vi "_API_BINANCE_GET_SystemStatus.vi"(0 "BinanceAPI in":refnum<class "BinanceAPI_.lvclass">, 11 "error in (no error)":errorcluster) -> (4 "BinanceAPI out":refnum<class "BinanceAPI_.lvclass">, 6 "systemStatus ok? (if True  all work normaly)":bool, 14 "Body":string, 15 "error out":errorcluster)   [LabVIEW 2022 SP3, in "BinanceAPI_.lvclass"]
doc: "https://binance-docs.github.io/apidocs/spot/en/#system-status-system"
uses:
  BinanceAPI_.lvclass
  BinanceAPI_.lvclass/BinanceAPI_.ctl
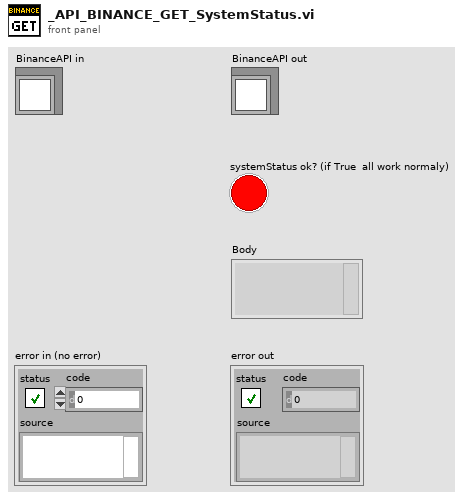
[diagram p1: front panel]
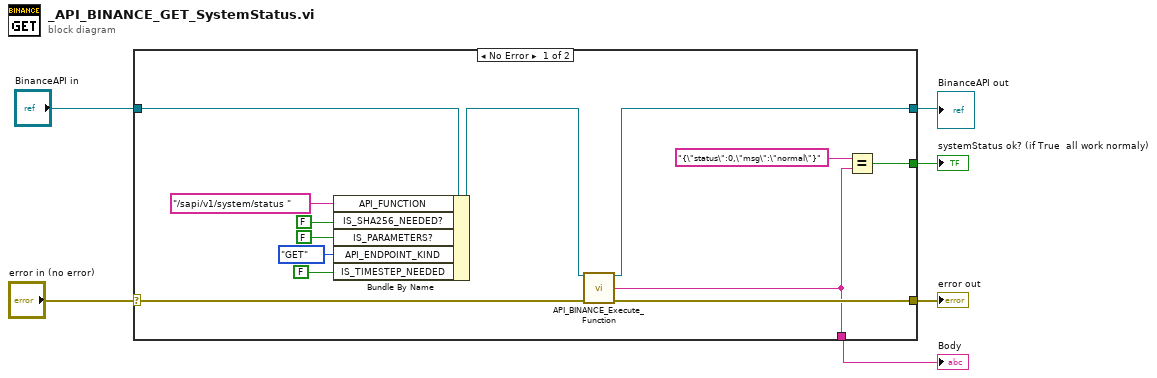
[diagram p0: block diagram]
diagram:
  n1 = case shown="No Error" "error in (no error)" {
    selector: "error in (no error)" -> [w12 w21]
    tunnel: [w11 w21] -> w5
    tunnel: [w13 w20] -> w1
    tunnel: "BinanceAPI in" -> [w19 w20]
    tunnel: [w8 _] -> w4
    tunnel: [w7 _] -> w3
    frame No Error {
      n2 = Bundle By Name(cluster=w19, "API_FUNCTION"="/sapi/v1/system/status ", "IS_SHA256_NEEDED?"=FALSE, "IS_PARAMETERS?"=FALSE, "API_ENDPOINT_KIND"=enum16{"POST", "DELETE", "GET", "PUT"}."GET", "IS_TIMESTEP_NEEDED"=FALSE) -> (w14:refnum<class "BinanceAPI_.lvclass">)
      n3 = call "API_BINANCE_Execute_Function.vi"("BinanceAPI in"=w14, "error in (no error)"=w12) -> ("BinanceAPI out"=w13:refnum<class "BinanceAPI_.lvclass">, "Body"=w7:string, "error out"=w11:errorcluster)  [unwired: 9 in, 2 out]
      n4 = Equal?(x="{\"status\":0,\"msg\":\"normal\"}", y=w7) -> (x = y?=w8:bool)
    }
    frame Error {
    }
  }
  "error out" <- w5
  "systemStatus ok? (if True  all work normaly)" <- w4
  "Body" <- w3
  "BinanceAPI out" <- w1
